vi "Class.SaveCtrls.Load.vi"(8 "error in":errorcluster, 11 "Save Control States in":refnum<class "Class.SaveCtrls.lvclass">) -> (0 "error out":errorcluster, 3 "Save Control States out":refnum<class "Class.SaveCtrls.lvclass">)   [LabVIEW 2024, in "EQMF.lvlib" / "Config Utils.lvlib" / "Class.SaveCtrls.lvclass"]
uses:
  Class.SaveCtrls.lvclass
  Class.SaveCtrls.lvclass/Class.SaveCtrls.ctl
  Files/File Utils.lvlib
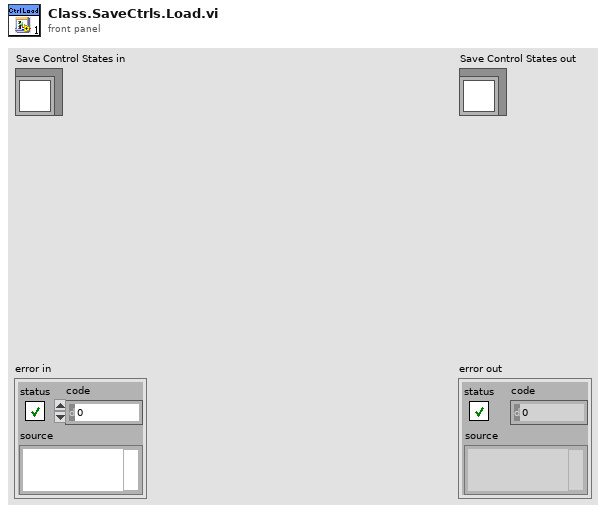
[diagram p1: front panel]
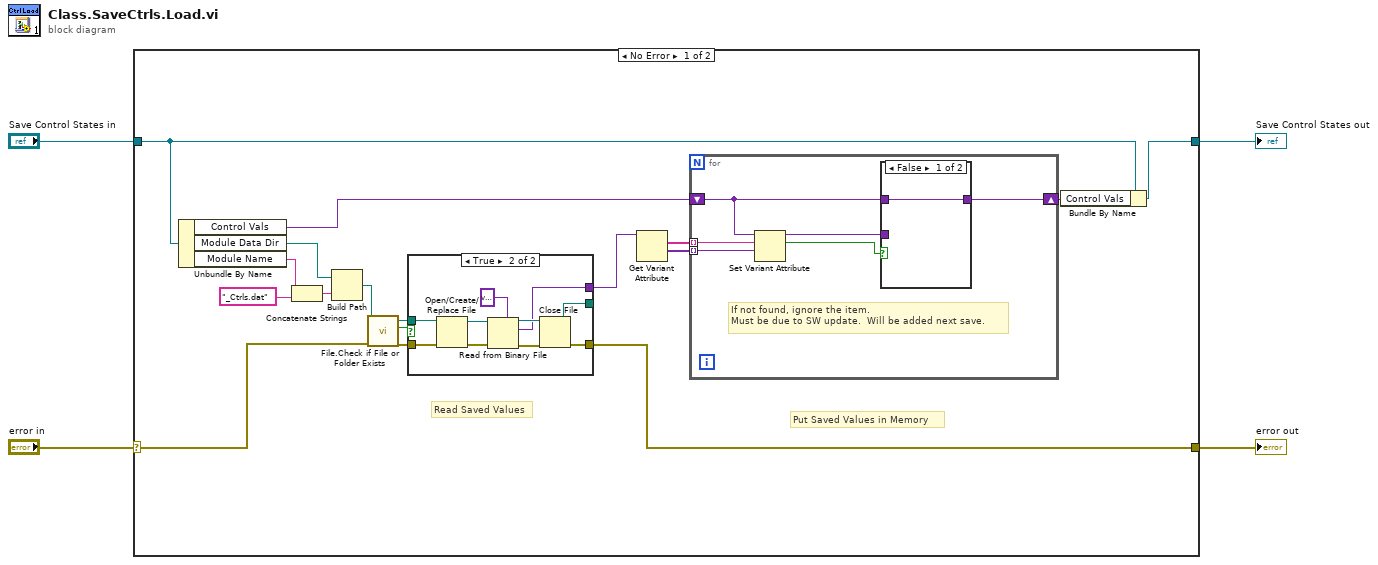
[diagram p0: block diagram]
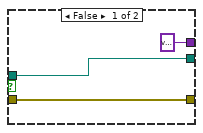
[diagram p3: hidden frame]
diagram:
  n1 = case shown="No Error" "error in" {
    selector: "error in" -> [w21 w44]
    tunnel: [w19 w44] -> w3
    tunnel: [w18 w43] -> w1
    tunnel: "Save Control States in" -> [w20 w43]
    frame No Error {
      # "Put Saved Values in Memory"
      # "Read Saved Values"
      n2 = Unbundle By Name(w20) -> ("Control Vals"=w6:variant, "Module Data Dir"=w11:path, "Module Name"=w10:string)
      n3 = Concatenate Strings(w10, "_Ctrls.dat") -> (w13:string)
      n4 = Build Path(base path=w11, name or relative path=w13) -> (appended path=w17:path)
      n5 = call "File.Check if File or Folder Exists.vi"("error in"=w21, "Path"=w17) -> ("error out"=w16:errorcluster, "Exists"=w14:bool, "Dup Path"=w15:path)  [unwired: 5 in, 2 out]
      n6 = case shown="True" w14 {
        tunnel: w16 -> [w30 w42]
        tunnel: w15 -> [w31 w41]
        tunnel: [w31 w36] -> _
        tunnel: [variant ("variant") w34] -> w7
        tunnel: [w30 w33] -> w19
        frame False {
        }
        frame True {
          n7 = Open/Create/Replace File(file path (use dialog)=w41, error in=w42) -> (refnum out=w40:refnum<file>, error out=w39:errorcluster)  [unwired: 4 in, 1 out]
          n8 = Read from Binary File(5:variant ("variant"), 8:w39, 11:w40) -> (0:w37:errorcluster, 2:w34:variant, 3:w38:refnum<file>)  [unwired: 3 in, 1 out]
          n9 = Close File(refnum=w38, error in=w37) -> (path=w36:path, error out=w33:errorcluster)
        }
      }
      n10 = Get Variant Attribute(Variant=w7) -> (names=w8:string[], values=w9:variant[])  [unwired: 3 in, 2 out]
      n11 = for {
        tunnel: w8 -> [w27] mode=indexing
        tunnel: w9 -> [w26] mode=indexing
        shift-right: [w23] -> w5
        shift-left: w6 -> [w24]
        # "If not found, ignore the item.\nMust be due to SW update.  Will be added next save."
        n12 = Set Variant Attribute(Variant=w24, name=w27, value=w26) -> (Variant out=w25:variant, replaced=w22:bool)  [unwired: 1 in, 1 out]
        n13 = case shown="False" w22 {
          tunnel: w25 -> [_ w29]
          tunnel: w24 -> [w28 _]
          tunnel: [w28 w29] -> w23
          frame False {
          }
          frame True {
          }
        }
      }
      n14 = Bundle By Name(cluster=w20, "Control Vals"=w5) -> (w18:refnum<class "Class.SaveCtrls.lvclass">)
    }
    frame Error {
    }
  }
  "error out" <- w3
  "Save Control States out" <- w1
